vi "Verify Shared Binary Versions.vi"() -> ()   [LabVIEW 2020, in "examples.lvlib"]
uses:
  examples.lvlib
  common/Library Name.ctl
  6ec88621-6f7e-4f72-ae85-70473001582e.vi
  <vilib>/Utility/error.llb/Error Cluster From Error Code.vi
  common/common.lvlib
  image/image.lvlib
  video_io/video_io.lvlib
  feature_detection/feature_detection.lvlib
  ar/ar.lvlib
  feature_detection/Text Tesseract/Text Tesseract.lvclass
panel:
  out "Result":cluster{"Info":string, "OK":bool}[](array[cluster])
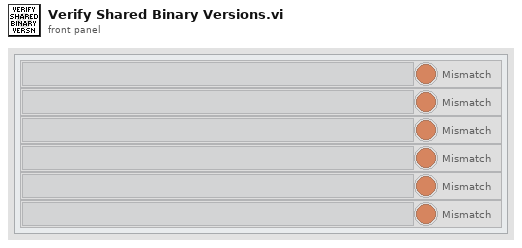
[diagram p1: front panel]
types:
  T1 = typedef "common.lvlib/Library Name.ctl" = enum16{"Core", "Feature Detection", "Augmented Reality", "DNN", "Tesseract", "Video IO"}
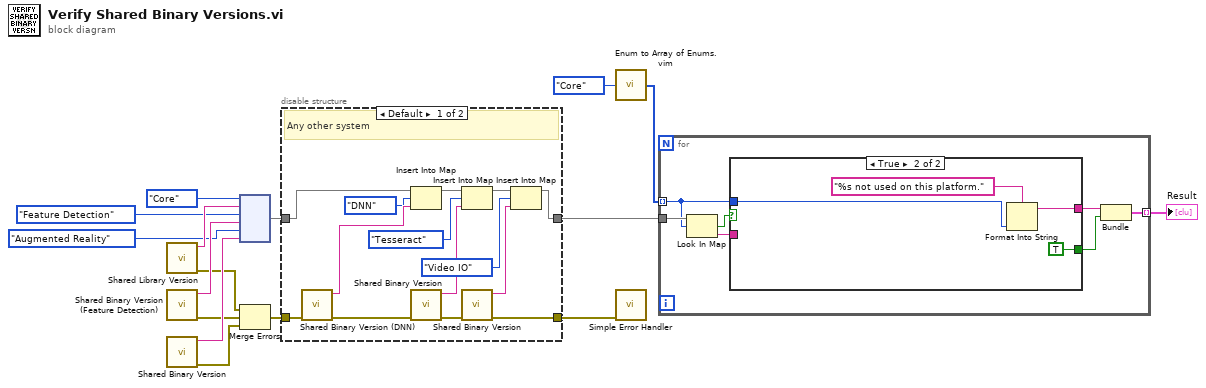
[diagram p0: block diagram]
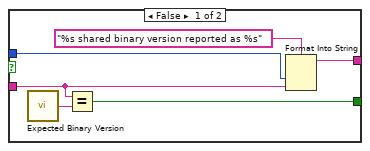
[diagram p2: hidden frame]
diagram:
  n1 = call "Shared Library Version.vi"() -> ("error out"=w9:errorcluster, "Version"=w15:string)  [unwired: 10 in]
  n2 = call "Shared Binary Version (Feature Detection).vi"() -> ("error out"=w8:errorcluster, "Version"=w14:string)  [unwired: 10 in]
  n3 = call "Shared Binary Version.vi"() -> ("error out"=w7:errorcluster, "Version"=w12:string)  [unwired: 10 in]
  n4 = node(Library_Name."Core" ("Library"), w15, Library_Name."Feature Detection" ("key"), w14, Library_Name."Augmented Reality" ("key"), w12) -> (w10:map{T1, string})
  n5 = Merge Errors(w9, w8, w7) -> (w6:errorcluster)
  n6 = disable-structure shown="Default" {
    disable-tunnel: [w24 w32] -> w5
    disable-tunnel: w10 -> [w30 w32]
    disable-tunnel: w6 -> [w22 w31]
    disable-tunnel: [w17 w31] -> w2
    frame condition #0 (active) {
      # "Any other system"
      n7 = call "Shared Binary Version (DNN).vi"("error in (no error)"=w22) -> ("error out"=w21:errorcluster, "Version"=w29:string)  [unwired: 9 in]
      n8 = Insert Into Map(map in=w30, key=Library_Name."DNN", value=w29) -> (map out=w27:map{T1, string})  [unwired: 2 out]
      n9 = call "Shared Binary Version.vi"("error in (no error)"=w21) -> ("error out"=w20:errorcluster, "Version"=w26:string)  [unwired: 9 in]
      n10 = Insert Into Map(map in=w27, key=Library_Name."Tesseract", value=w26) -> (map out=w25:map{T1, string})  [unwired: 2 out]
      n11 = call "Shared Binary Version.vi"("error in (no error)"=w20) -> ("error out"=w17:errorcluster, "Version"=w23:string)  [unwired: 9 in]
      n12 = Insert Into Map(map in=w25, key=Library_Name."Video IO", value=w23) -> (map out=w24:map{T1, string})  [unwired: 2 out]
    }
    frame condition #1 {
      # "ARM 32 RT Target (myRIO, LINX...)"
    }
  }
  n13 = call "Enum to Array of Enums.vim"("enum"=Library_Name."Core" ("Library")) -> ("array of enums"=w3:T1[])
  n14 = call <vilib>:"Simple Error Handler.vi"("error in (no error)"=w2) -> ()  [unwired: 4 in, 5 out]
  n15 = for {
    tunnel: w5 -> [w39]
    tunnel: w3 -> [w36] mode=indexing
    tunnel: [w33] -> w1 mode=indexing
    n16 = Look In Map(map=w39, key=w36) -> (key not found?=w38:bool, value=w37:string)  [unwired: 1 in]
    n17 = case shown="True" w38 {
      tunnel: [w44 w48] -> w35
      tunnel: w37 -> [w41 _]
      tunnel: w36 -> [w43 w49]
      tunnel: [w40 TRUE] -> w34
      frame False {
        n18 = call "Expected Binary Version.vi"() -> ("Expected Version"=w42:string)
        n19 = Equal?(x=w41, y=w42) -> (x = y?=w40:bool)
        n20 = Format Into String(format string="%s shared binary version reported as %s", w43, w41) -> (resulting string=w44:string)  [unwired: 2 in, 1 out]
      }
      frame True {
        n21 = Format Into String(format string="%s not used on this platform.", w49) -> (resulting string=w48:string)  [unwired: 2 in, 1 out]
      }
    }
    n22 = Bundle(w35, w34) -> (w33:cluster{string, bool})  [unwired: 1 in]
  }
  "Result" <- w1
